vi "tearDown.vi"(8 "error in (no error)":errorcluster, 11 "reference in":refnum<class "SLSC Switch Scripting System Tests.lvclass">=refnum) -> (0 "error out":errorcluster, 3 "reference out":refnum<class "SLSC Switch Scripting System Tests.lvclass">)   [LabVIEW 2017, in "SLSC Switch Scripting System Tests.lvclass"]
doc: "tearDown runs after the test method has completed. Use this method to clean up any operations or references that were opened by setUp or the test method. Unit tests should be independent of other unit tests so this VI should ensure that the next test can run in a 'clean' test environment."
uses:
  SLSC Switch Scripting System Tests.lvclass
  SLSC Switch Scripting System Tests.lvclass/SLSC Switch Scripting System Tests.ctl
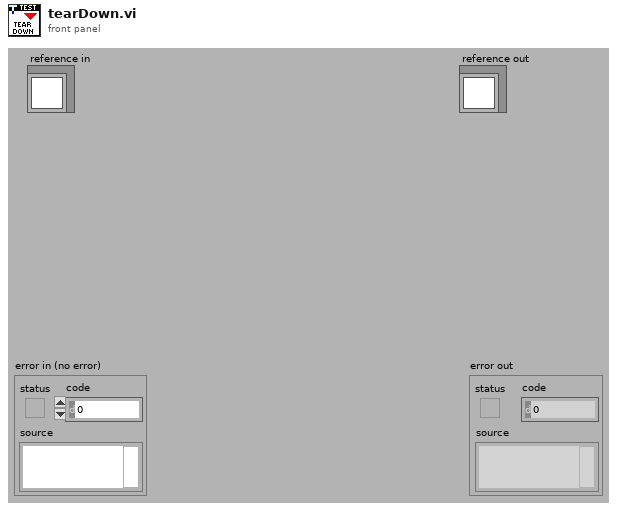
[diagram p1: front panel]
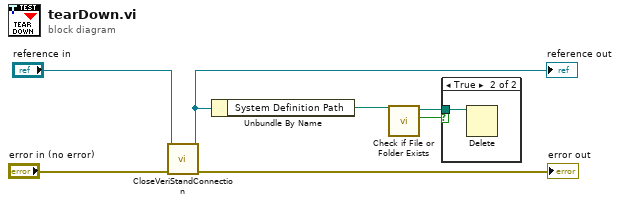
[diagram p0: block diagram]
diagram:
  n1 = call-dynamic "CloseVeriStandConnection.vi"("error in (no error)"="error in (no error)", "VeriStand Test Case in"="reference in") -> ("error out"=→"error out":errorcluster, "VeriStand Test Case out"=w4:refnum<class "SLSC Switch Scripting System Tests.lvclass">)  [unwired: 8 in]
  "reference out" <- w4
  n2 = Unbundle By Name(w4) -> ("System Definition Path"=w3:path)
  n3 = call <vilib>:"Check if File or Folder Exists.vi"("path"=w3) -> ("file or folder exists?"=w2:bool, "dup path"=w1:path)  [unwired: 8 in, 1 out]
  n4 = case shown="True" w2 {
    tunnel: w1 -> [_ w8]
    frame False {
    }
    frame True {
      n5 = Delete(path (use dialog)=w8) -> ()  [unwired: 4 in, 3 out]
    }
  }
